vi "Clean Visa Errors.vi"(8 "error in (no error)":errorcluster, 11 "VisaComms in":refnum<class "VisaComms.lvclass">) -> (0 "error out":errorcluster, 3 "VisaComms out":refnum<class "VisaComms.lvclass">)   [LabVIEW 2024, in "CTI.lvlib" / "VisaComms.lvclass"]
uses:
  VisaComms.lvclass
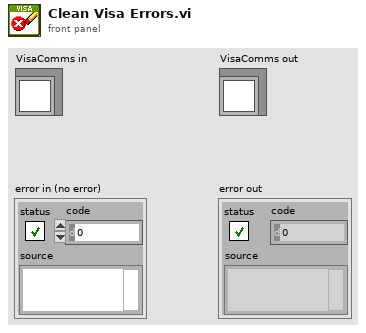
[diagram p1: front panel]
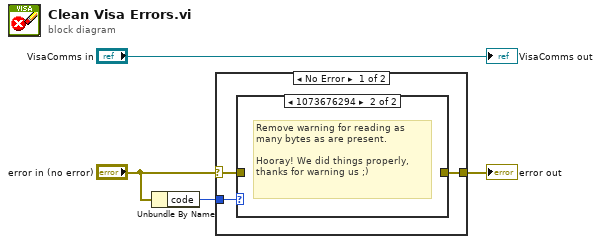
[diagram p0: block diagram]
diagram:
  n1 = Unbundle By Name("error in (no error)") -> ("code"=w4:i32)
  n2 = case shown="No Error" "error in (no error)" {
    selector: "error in (no error)" -> [w6 w9]
    tunnel: w4 -> [w7 _]
    tunnel: [w5 w9] -> w2
    frame No Error {
      n3 = case shown="1073676294" w7 {
        tunnel: w6 -> [w8 _]
        tunnel: [w8 _] -> w5
        frame Default {
        }
        frame 1073676294 {
          # "Remove warning for reading as many bytes as are present.\n\nHooray! We did things properly, thanks for warning us ;)"
        }
      }
    }
    frame Error {
    }
  }
  "error out" <- w2
  "VisaComms out" <- "VisaComms in"
